vi "HW3_2017_WMA.vi"() -> ()   [LabVIEW 2017]
panel:
  out "Boolean 3":bool
  out "Boolean 2":bool
  out "Cluster 2":T1
  out "Cluster 3":T1
  out "Cluster 4":T1
  out "Cluster 5":T1
  out "Cluster 6":T1
  out "Cluster 7":T1
  in  "START/STOP/CLEAR":bool
  in  "Path":path
  in  "min":dbl
  in  "hour":dbl
  in  "OK Button":bool
  out "Boolean":bool
  in  "SET ALARM":bool
  out "ALARMING TIME":string
  out "DATE":string
  in  "reinstate":bool
  in  "sec":dbl
  in  "min":dbl
  in  "hour":dbl
  in  "reset":bool
  out "sec":dbl(knob) scale=0.0..60.0
  out "min":dbl(knob) scale=0.0..60.0
  out "hour":dbl(knob) scale=0.0..12.0
  in  "stop":bool
  in  "OK Button 3":bool
  in  "Path 2":path
  out "new picture":picture
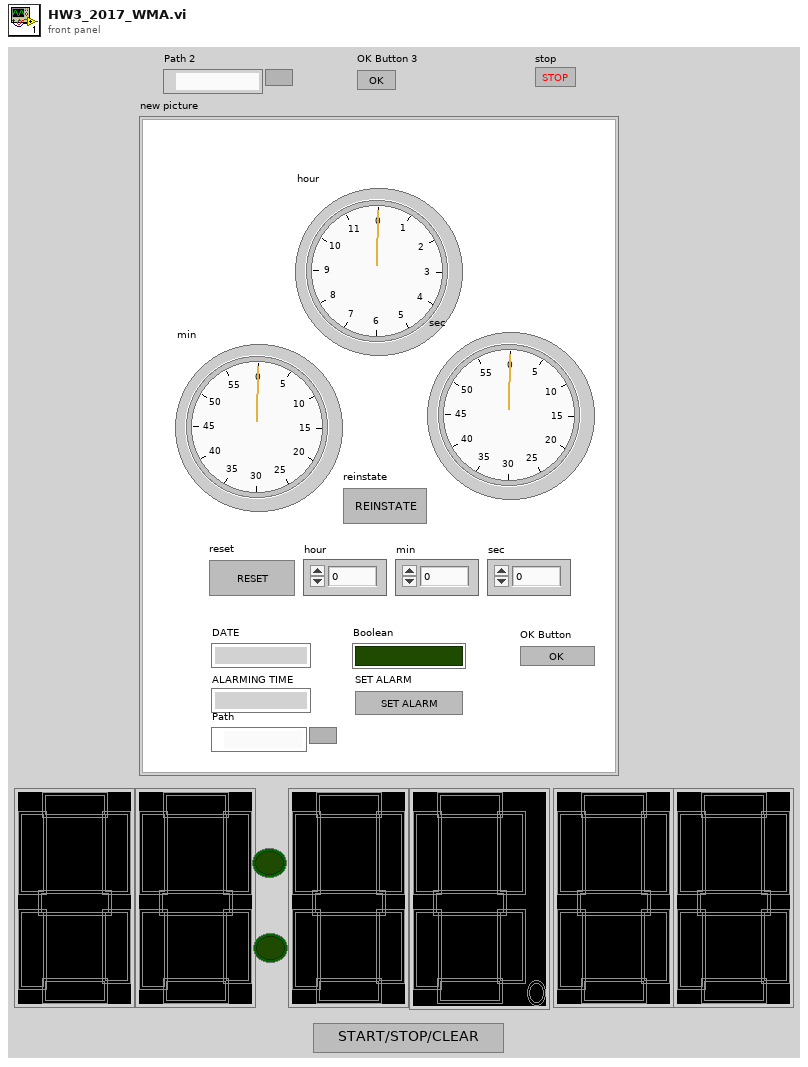
[diagram p1: front panel]
types:
  T1 = cluster{"0":bool, "1":bool, "2":bool, "3":bool, " 4":bool, "5":bool, "6":bool, "p":bool}
  T2 = cluster{"0":bool, "1":bool, "2":bool, "3":bool, " 4":bool, "5":bool, "6":bool, "p":bool}[]
  T3 = typedef "LVDateTimeRec.ctl" = cluster{"fractional second":dbl, "second":i32, "minute":i32, "hour":i32, "day of month":i32, "month":i32, "year":i32, "day of week":i32, "day of year":i32, "DST":i32}
  T4 = typedef "imagedata.ctl" = cluster{"image type":i32, "image depth":i32, "image":u8[], "mask":u8[], "colors":u32[], "Rectangle":cluster{"left":i16, "top":i16, "right":i16, "bottom":i16}}
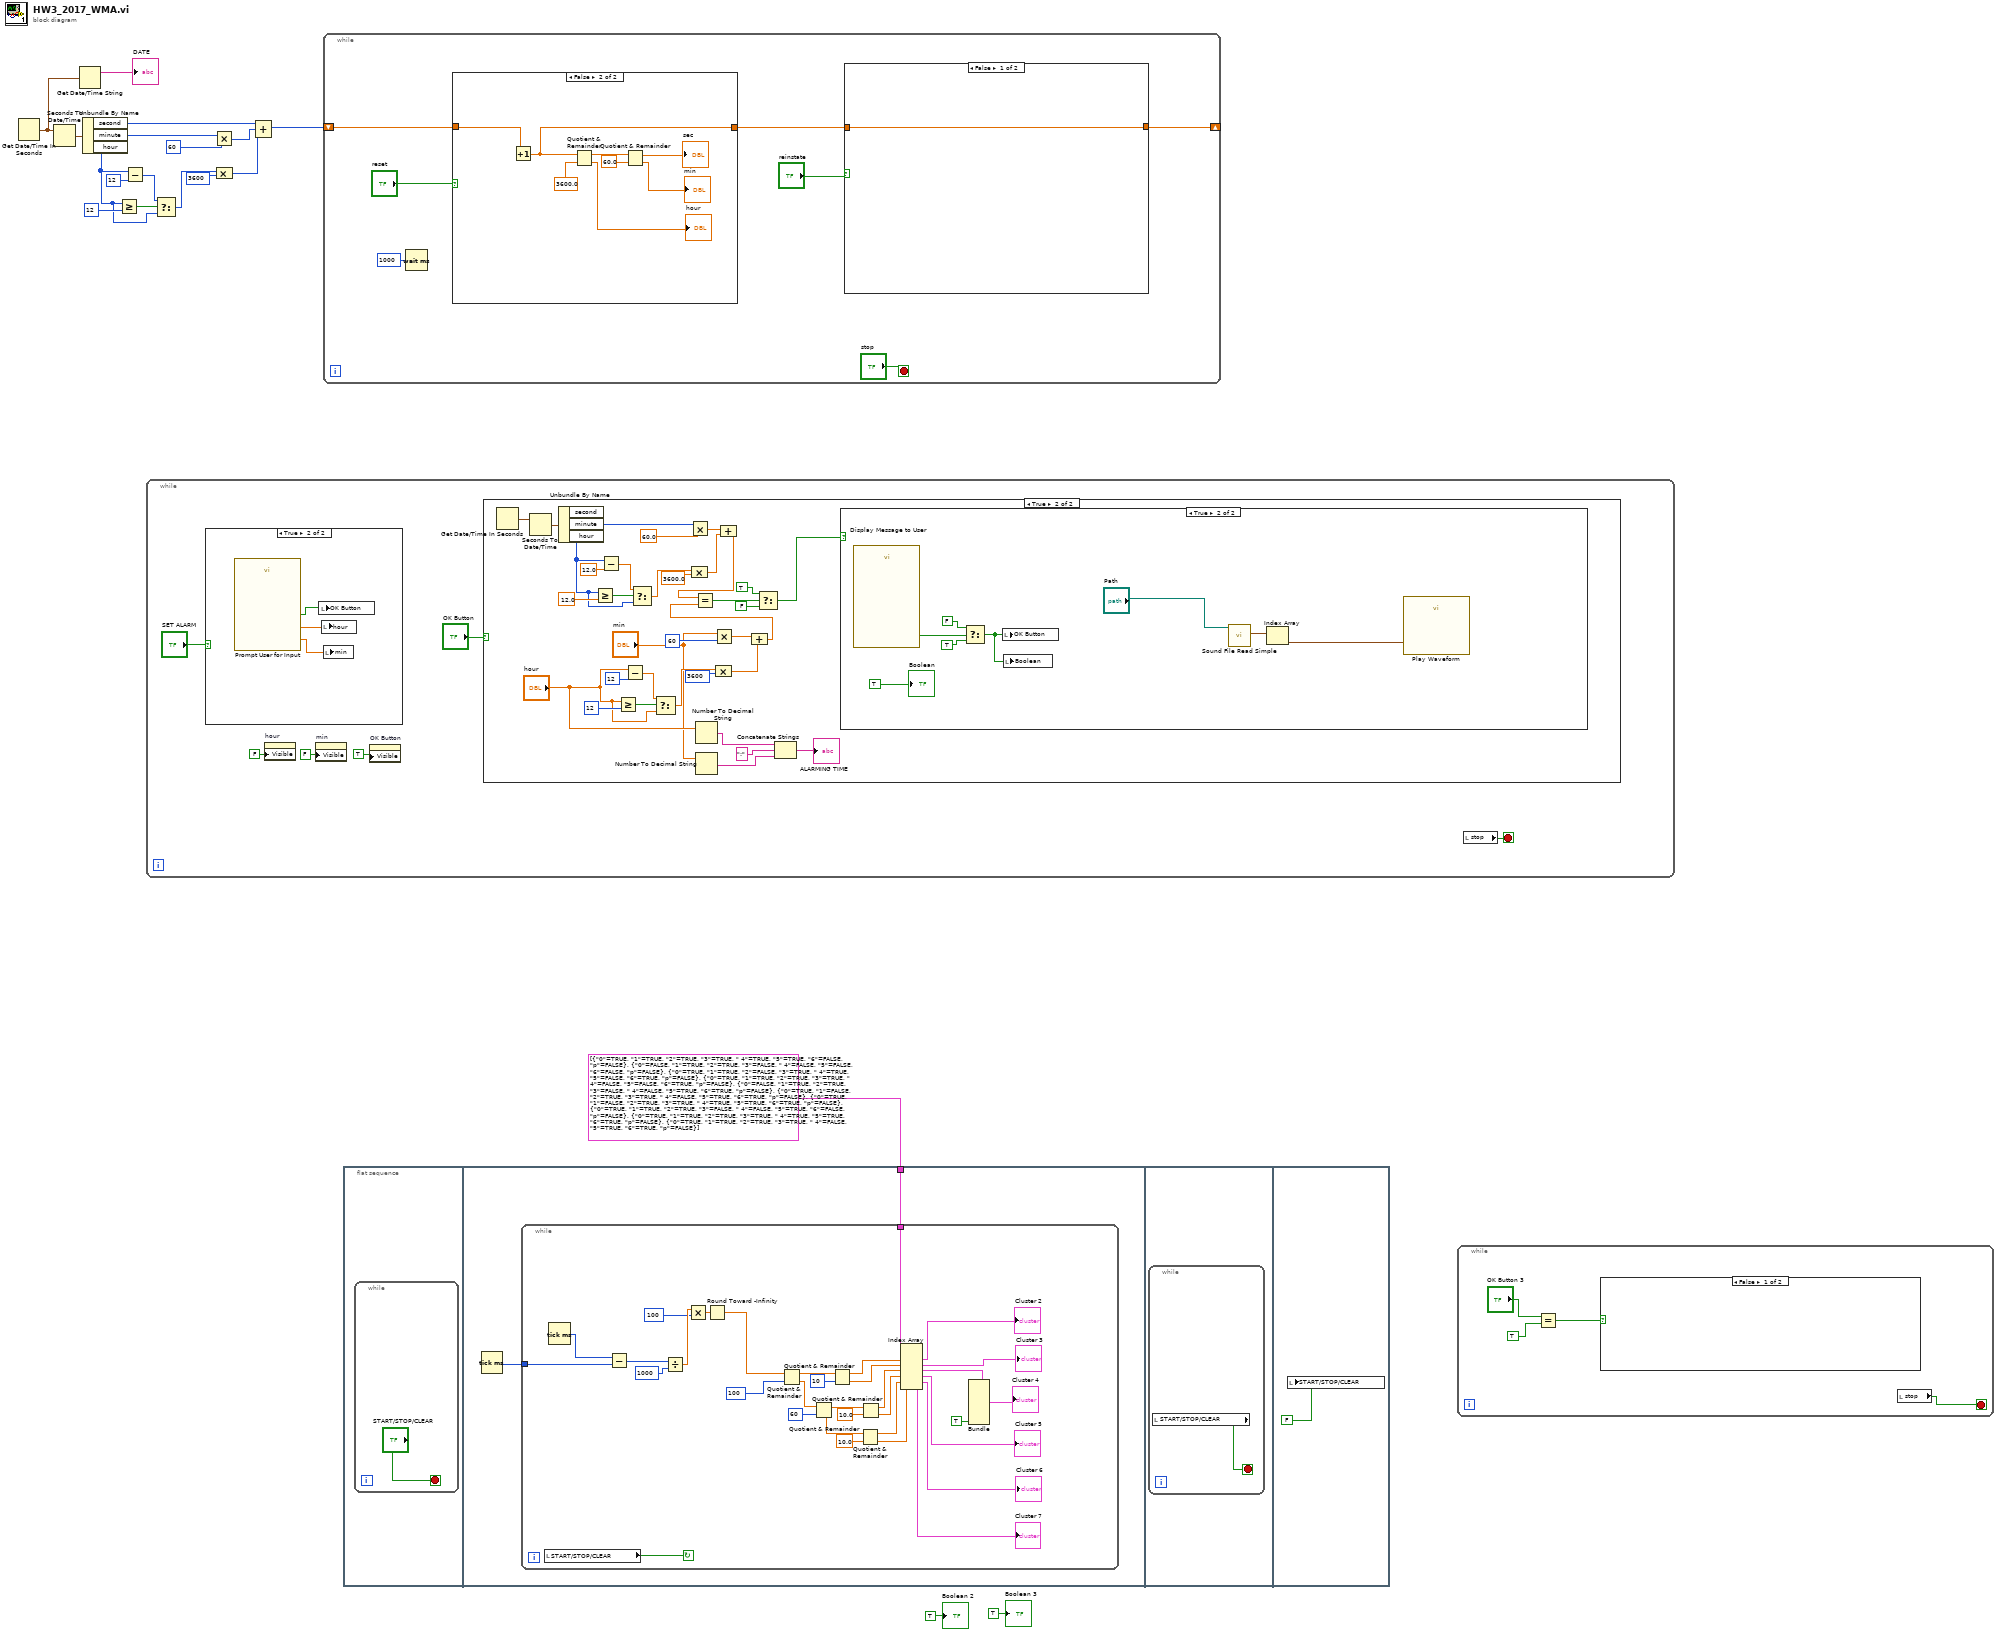
[diagram p0: block diagram]
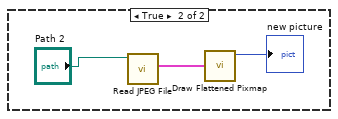
[diagram p2: hidden frame]
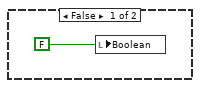
[diagram p4: hidden frame]
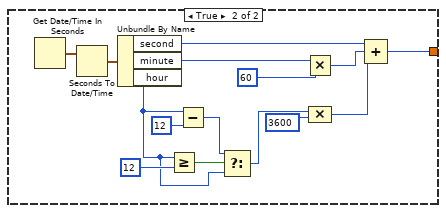
[diagram p6: hidden frame]
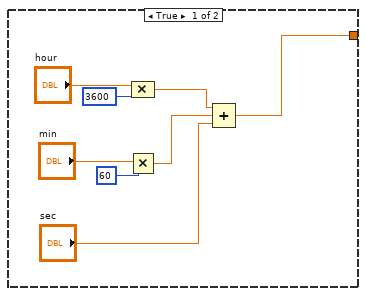
[diagram p7: hidden frame]
diagram:
  n1 = Get Date/Time In Seconds() -> (seconds since 1Jan1904=w8:timestamp)
  n2 = Seconds To Date/Time(time stamp (now)=w8) -> (date time rec=w17:T3)  [unwired: 1 in]
  n3 = Get Date/Time String(seconds (now)=w8) -> (date string=→"DATE":string)  [unwired: 2 in, 1 out]
  n4 = Unbundle By Name(w17) -> ("second"=w15:i32, "minute"=w16:i32, "hour"=w10:i32)
  n5 = Greater Or Equal?(x=w10, y=12) -> (x >= y?=w13:bool)
  n6 = Subtract(x=w10, y=12) -> (x-y=w11:i32)
  n7 = while {
    stop <- w21 stop-if-true
    n8 = case shown="True" "SET ALARM" {
      frame False {
      }
      frame True {
        n9 = call "Prompt User for Input"() -> ("Minute"=w71:dbl, "Hour"=w70:dbl, "OK"=w69:bool)  [unwired: 16 in, 1 out]
        n10 = local write "OK Button"(w69) -> ()
        n11 = local write "hour"(w70) -> ()
        n12 = local write "min"(w71) -> ()
      }
    }
    n13 = property on="hour" class="DigNum (strict)"("Visible"=FALSE) -> ()  [unwired: 2 in, 2 out]
    n14 = property on="min" class="DigNum (strict)"("Visible"=FALSE) -> ()  [unwired: 2 in, 2 out]
    n15 = property on="OK Button" class="Bool (strict)"("Visible"=TRUE) -> ()  [unwired: 2 in, 2 out]
    n16 = case shown="True" "OK Button" {
      frame False {
      }
      frame True {
        n17 = Get Date/Time In Seconds() -> (seconds since 1Jan1904=w29:timestamp)
        n18 = Seconds To Date/Time(time stamp (now)=w29) -> (date time rec=w32:T3)  [unwired: 1 in]
        n19 = Unbundle By Name(w32) -> ("minute"=w33:i32, "hour"=w27:i32)  [unwired: 1 out]
        n20 = Greater Or Equal?(x=w27, y=12.0) -> (x >= y?=w35:bool)
        n21 = Subtract(x=w27, y=12.0) -> (x-y=w37:dbl)
        n22 = Greater Or Equal?(x="hour", y=12) -> (x >= y?=w54:bool)
        n23 = Subtract(x="hour", y=12) -> (x-y=w52:dbl)
        n24 = Select(t=w37, s=w35, f=w27) -> (s? t:f=w38:dbl)
        n25 = Select(t=w52, s=w54, f="hour") -> (s? t:f=w51:dbl)
        n26 = Multiply(x=w33, y=60.0) -> (x*y=w39:dbl)
        n27 = Compound Arithmetic op=MULTIPLY(w38, 3600.0) -> (w40:dbl)
        n28 = Number To Decimal String(number="hour") -> (decimal integer string=w46:string)  [unwired: 1 in]
        n29 = Number To Decimal String(number="min") -> (decimal integer string=w44:string)  [unwired: 1 in]
        n30 = Multiply(x="min", y=60) -> (x*y=w57:dbl)
        n31 = Compound Arithmetic op=MULTIPLY(w51, 3600) -> (w56:dbl)
        n32 = Compound Arithmetic op=ADD(w39, w40) -> (w28:dbl)
        n33 = Compound Arithmetic op=ADD(w57, w56) -> (w50:dbl)
        n34 = Equal?(x=w28, y=w50) -> (x = y?=w49:bool)
        n35 = Select(t=TRUE, s=w49, f=FALSE) -> (s? t:f=w26:bool)
        n36 = Concatenate Strings(w46, ":", w44) -> (→"ALARMING TIME":string)
        n37 = case shown="True" w26 {
          frame False {
            n38 = local write "Boolean"(FALSE ("Boolean")) -> ()
          }
          frame True {
            n39 = call "Display Message to User"() -> ("OK"=w66:bool)  [unwired: 10 in, 1 out]
            n40 = Select(t=FALSE ("Boolean"), s=w66, f=TRUE) -> (s? t:f=w64:bool)
            n41 = local write "OK Button"(w64) -> ()
            n42 = local write "Boolean"(w64) -> ()
            n43 = call <vilib>:"Sound File Read Simple.vi"("path"="Path") -> ("data"=w61:waveform(dbl)[])  [unwired: 7 in, 3 out]
            n44 = Index Array(array=w61) -> (element=w62:waveform(dbl))  [unwired: 1 in]
            n45 = call "Play Waveform"("Data"=w62) -> ()  [unwired: 18 in, 1 out]
            "Boolean" <- TRUE ("Boolean")
          }
        }
      }
    }
    n46 = local read "stop"() -> (w21:bool)
  }
  n47 = Select(t=w11, s=w13, f=w10) -> (s? t:f=w9:i32)
  n48 = Multiply(x=w16, y=60) -> (x*y=w5:i32)
  n49 = Compound Arithmetic op=MULTIPLY(w9, 3600) -> (w4:i32)
  n50 = Compound Arithmetic op=ADD(w15, w5, w4) -> (w7:i32)
  n51 = while {
    shift-right: [w73] -> _
    shift-left: w7 -> [w77]
    stop <- "stop" stop-if-true
    n52 = Wait (ms)(milliseconds to wait=u32 1000) -> ()  [unwired: 1 out]
    n53 = case shown="False" "reset" {
      tunnel: w77 -> [_ w110]
      tunnel: [w95 w103] -> w74
      frame True {
        n54 = Multiply(x="min", y=60) -> (x*y=w97:dbl)
        n55 = Compound Arithmetic op=MULTIPLY("hour", 3600) -> (w98:dbl)
        n56 = Compound Arithmetic op=ADD(w98, w97, "sec") -> (w95:dbl)
      }
      frame False {
        n57 = Increment(x=w110) -> (x+1=w103:dbl)
        n58 = Quotient & Remainder(x=w103, y=3600.0) -> (x-y*floor(x/y)=w108:dbl, floor(x/y)=→"hour":dbl)
        n59 = Quotient & Remainder(x=w108, y=60.0) -> (x-y*floor(x/y)=→"sec":dbl, floor(x/y)=→"min":dbl)
      }
    }
    n60 = case shown="False" "reinstate" {
      tunnel: w74 -> [w79 _]
      tunnel: [w79 w80] -> w73
      frame False {
      }
      frame True {
        n61 = Get Date/Time In Seconds() -> (seconds since 1Jan1904=w91:timestamp)
        n62 = Seconds To Date/Time(time stamp (now)=w91) -> (date time rec=w90:T3)  [unwired: 1 in]
        n63 = Unbundle By Name(w90) -> ("second"=w87:i32, "minute"=w89:i32, "hour"=w82:i32)
        n64 = Greater Or Equal?(x=w82, y=12) -> (x >= y?=w85:bool)
        n65 = Subtract(x=w82, y=12) -> (x-y=w83:i32)
        n66 = Select(t=w83, s=w85, f=w82) -> (s? t:f=w81:i32)
        n67 = Multiply(x=w89, y=60) -> (x*y=w92:i32)
        n68 = Compound Arithmetic op=MULTIPLY(w81, 3600) -> (w88:i32)
        n69 = Compound Arithmetic op=ADD(w87, w92, w88) -> (w80:i32)
      }
    }
  }
  n70 = flat-sequence {
    tunnel: T2 [{"0"=TRUE, "1"=TRUE, "2"=TRUE, "3"=TRUE, " 4"=TRUE, "5"=TRUE, "6"=FALSE, "p"=FALSE}, {"0"=FALSE, "1"=TRUE, "2"=TRUE, "3"=FALSE, " 4"=FALSE, "5"=FALSE, "6"=FALSE, "p"=FALSE}, {"0"=TRUE, "1"=TRUE, "2"=FALSE, "3"=TRUE, " 4"=TRUE, "5"=FALSE, "6"=TRUE, "p"=FALSE}, {"0"=TRUE, "1"=TRUE, "2"=TRUE, "3"=TRUE, " 4"=FALSE, "5"=FALSE, "6"=TRUE, "p"=FALSE}, {"0"=FALSE, "1"=TRUE, "2"=TRUE, "3"=FALSE, " 4"=FALSE, "5"=TRUE, "6"=TRUE, "p"=FALSE}, {"0"=TRUE, "1"=FALSE, "2"=TRUE, "3"=TRUE, " 4"=FALSE, "5"=TRUE, "6"=TRUE, "p"=FALSE}, {"0"=TRUE, "1"=FALSE, "2"=TRUE, "3"=TRUE, " 4"=TRUE, "5"=TRUE, "6"=TRUE, "p"=FALSE}, {"0"=TRUE, "1"=TRUE, "2"=TRUE, "3"=FALSE, " 4"=FALSE, "5"=TRUE, "6"=FALSE, "p"=FALSE}, {"0"=TRUE, "1"=TRUE, "2"=TRUE, "3"=TRUE, " 4"=TRUE, "5"=TRUE, "6"=TRUE, "p"=FALSE}, {"0"=TRUE, "1"=TRUE, "2"=TRUE, "3"=TRUE, " 4"=FALSE, "5"=TRUE, "6"=TRUE, "p"=FALSE}] -> [w112]
    frame #0 {
      n71 = while {
        stop <- "START/STOP/CLEAR" stop-if-true
      }
    }
    frame #1 {
      n72 = Tick Count (ms)() -> (millisecond timer value=w113:u32)
      n73 = while {
        tunnel: w113 -> [w145]
        tunnel: w112 -> [w127]
        stop <- w142 continue-if-true
        n74 = local read "START/STOP/CLEAR"() -> (w142:bool)
        n75 = Tick Count (ms)() -> (millisecond timer value=w146:u32)
        n76 = Subtract(x=w146, y=w145) -> (x-y=w144:u32)
        n77 = Divide(x=w144, y=1000) -> (x/y=w141:dbl)
        n78 = Multiply(x=w141, y=100) -> (x*y=w139:dbl)
        n79 = Round Toward -Infinity(1:w139) -> (0:w126:dbl)
        n80 = Quotient & Remainder(x=w126, y=100) -> (x-y*floor(x/y)=w133:dbl, floor(x/y)=w123:dbl)
        n81 = Quotient & Remainder(x=w123, y=60) -> (x-y*floor(x/y)=w120:dbl, floor(x/y)=w116:dbl)
        n82 = Quotient & Remainder(x=w133, y=10) -> (x-y*floor(x/y)=w134:dbl, floor(x/y)=w135:dbl)
        n83 = Quotient & Remainder(x=w116, y=10.0) -> (x-y*floor(x/y)=w115:dbl, floor(x/y)=w114:dbl)
        n84 = Quotient & Remainder(x=w120, y=10.0) -> (x-y*floor(x/y)=w119:dbl, floor(x/y)=w118:dbl)
        n85 = Index Array(array=w127, index #1=w134, index #2=w135, index #3=w119, index #4=w118, index #5=w115, index #6=w114) -> (element #1=→"Cluster 2":T1, element #2=→"Cluster 3":T1, element #3=w136:T1, element #4=→"Cluster 5":T1, element #5=→"Cluster 6":T1, element #6=→"Cluster 7":T1)
        n86 = Bundle(cluster=w136, "p"=TRUE) -> (→"Cluster 4":T1)  [unwired: 7 in]
      }
    }
    frame #2 {
      n87 = while {
        stop <- w147 stop-if-true
        n88 = local read "START/STOP/CLEAR"() -> (w147:bool)
      }
    }
    frame #3 {
      n89 = local write "START/STOP/CLEAR"(FALSE ("OK Button")) -> ()
    }
  }
  n90 = while {
    stop <- w149 stop-if-true
    n91 = Equal?(x="OK Button 3", y=TRUE) -> (x = y?=w150:bool)
    n92 = case shown="False" w150 {
      frame False {
      }
      frame True {
        n93 = call <vilib>:"Read JPEG File.vi"("path to JPEG file"="Path 2") -> ("image data"=w154:T4)  [unwired: 8 in, 2 out]
        n94 = call <vilib>:"Draw Flattened Pixmap.vi"("image data"=w154) -> ("new picture"=→"new picture":picture)  [unwired: 8 in]
      }
    }
    n95 = local read "stop"() -> (w149:bool)
  }
  "Boolean 2" <- TRUE ("Boolean")
  "Boolean 3" <- TRUE ("Boolean 2")
